vi "Waveforms To XY.vi"(8 "error in (no error)":errorcluster, 11 "AI Waveform":waveform(dbl)[](array[waveform])) -> (0 "error out":errorcluster, 3 "Array":cluster{dbl[], dbl[]}[](array[cluster]))   [LabVIEW 2016, in "Transport.lvclass"]
uses:
  Transport.lvclass
  <vilib>/Waveform/WDTOps.llb/WDT Waveform to XY Pairs DBL.vi
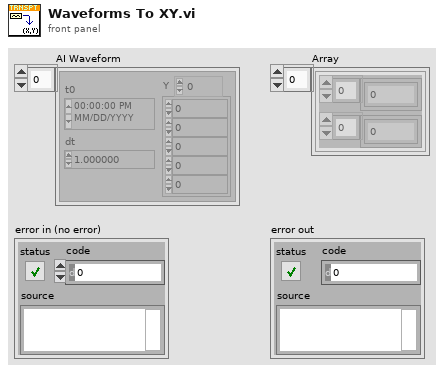
[diagram p1: front panel]
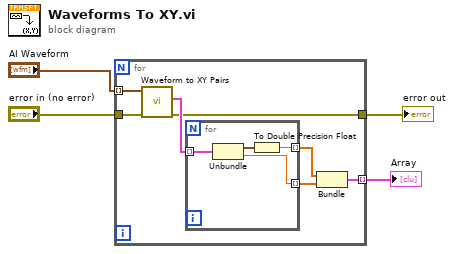
[diagram p0: block diagram]
diagram:
  n1 = for {
    tunnel: "AI Waveform" -> [w8] mode=indexing
    tunnel: "error in (no error)" -> [w11]
    tunnel: [w9] -> w2
    tunnel: [w5] -> w1 mode=indexing
    n2 = call-poly <vilib>:"Waveform to XY Pairs.vi"("error in (no error)"=w11, "waveform in"=w8) -> ("error out"=w9:errorcluster, "XY pairs"=w10:cluster{"x":timestamp, "y":dbl}[])  [unwired: 7 in, 1 out]
    n3 = for {
      tunnel: w10 -> [w15] mode=indexing
      tunnel: [w12] -> w7 mode=indexing
      tunnel: [w13] -> w6 mode=indexing
      n4 = Unbundle(w15) -> ("x"=w14:timestamp, "y"=w13:dbl)
      n5 = To Double Precision Float(number=w14) -> (double precision float=w12:dbl)
    }
    n6 = Bundle(w7, w6) -> (w5:cluster{dbl[], dbl[]})  [unwired: 1 in]
  }
  "error out" <- w2
  "Array" <- w1
